vi "wd_replaceAll (WFM).vi"(7 "WFM":waveform(dbl), 8 "error in (no error)":errorcluster, 9 "channel index":i32, 10 "data type":T7, 11 "meta in":T1={"TargetFile"=path "", "StreamMode"=enum."File", "Append?"=FALSE, "ChunkSize"=0, "TimeColumnMode"=enum."Empty", "TimestampFormat"="", "AbsoluteTime?"=FALSE, "FileAttribute "={"Creator"="", "Title"="", "SheetName"=""}, "Column"=[], "FileRef"=refnum, "MemoryRef"=[], "RecordInfo"=[], " ChannelPreviousInfo"=[], "ChannelFirstRecord"=[], "PredefinedFormattedValueLength"=20, "DiskTemplate"={"XMLRef"=[refnum, refnum, refnum, refnum, refnum, refnum], "ZipPath"=path "", "MetaFile"={"Ref"=refnum, "NextRow"=0, "NextPosition"=0, "Block"=[]}, "TempFolder"=path ""}}) -> (0 "error out":errorcluster, 3 "meta out":T1={"TargetFile"=path "", "StreamMode"=enum."File", "Append?"=FALSE, "ChunkSize"=0, "TimeColumnMode"=enum."Empty", "TimestampFormat"="", "AbsoluteTime?"=FALSE, "FileAttribute "={"Creator"="", "Title"="", "SheetName"=""}, "Column"=[], "FileRef"=refnum, "MemoryRef"=[], "RecordInfo"=[], " ChannelPreviousInfo"=[], "ChannelFirstRecord"=[], "PredefinedFormattedValueLength"=20, "DiskTemplate"={"XMLRef"=[refnum, refnum, refnum, refnum, refnum, refnum], "ZipPath"=path "", "MetaFile"={"Ref"=refnum, "NextRow"=0, "NextPosition"=0, "Block"=[]}, "TempFolder"=path ""}})   [LabVIEW 2017, in "NI_ExcelFile.lvlib"]
uses:
  <vilib>/express/express shared/NI_ExcelFile/NI_ExcelFile.lvlib
  <vilib>/express/express shared/NI_ExcelFile/Ctrls/DataType.ctl
  <vilib>/express/express shared/NI_ExcelFile/Ctrls/MainData.ctl
  <vilib>/express/express shared/NI_ExcelFile/Ctrls/StreamMode.ctl
  <vilib>/express/express shared/NI_ExcelFile/Ctrls/TimeColumnMode.ctl
  <vilib>/express/express shared/NI_ExcelFile/Ctrls/FileAttribute.ctl
  <vilib>/express/express shared/NI_ExcelFile/Ctrls/Columns.ctl
  <vilib>/express/express shared/NI_ExcelFile/Ctrls/ColumnInfo.ctl
  <vilib>/express/express shared/NI_ExcelFile/Ctrls/wd_recordInfo.ctl
  <vilib>/express/express shared/NI_ExcelFile/Ctrls/disk_TemplateFile.ctl
  <vilib>/express/express shared/NI_ExcelFile/Ctrls/meta_file.ctl
  <vilib>/express/express shared/NI_ExcelFile/Ctrls/meta_Block.ctl
  <vilib>/express/express shared/NI_ExcelFile/Ctrls/meta_BlockType.ctl
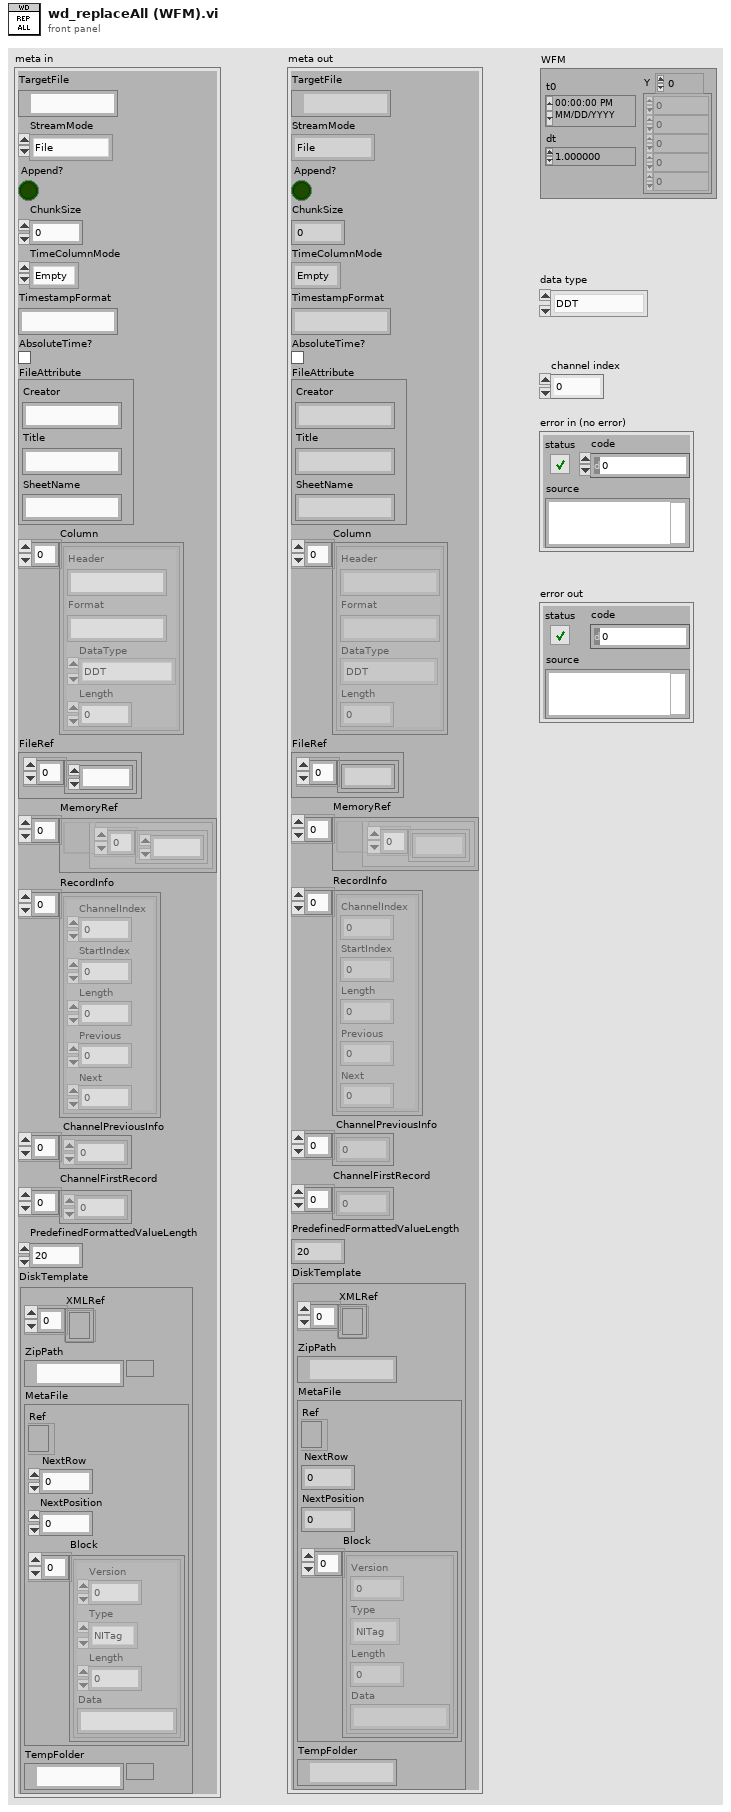
[diagram p1: front panel]
types:
  T1 = typedef "NI_ExcelFile.lvlib/MainData.ctl" = cluster{"TargetFile":path, "StreamMode":T2, "Append?":bool, "ChunkSize":u64, "TimeColumnMode":T3, "TimestampFormat":string, "AbsoluteTime?":bool, "FileAttribute ":T4, "Column":T5, "FileRef":refnum<k1>, "MemoryRef":refnum<data-value>[], "RecordInfo":T8[], " ChannelPreviousInfo":u32[], "ChannelFirstRecord":u32[], "PredefinedFormattedValueLength":i64, "DiskTemplate":T9}
  T2 = typedef "NI_ExcelFile.lvlib/StreamMode.ctl" = enum16{"File", "Memory"}
  T3 = typedef "NI_ExcelFile.lvlib/TimeColumnMode.ctl" = enum16{"Empty", "OnePerCh", "One"}
  T4 = typedef "NI_ExcelFile.lvlib/FileAttribute.ctl" = cluster{"Creator":string, "Title":string, "SheetName":string}
  T5 = typedef "NI_ExcelFile.lvlib/Columns.ctl" = T6[]
  T6 = typedef "NI_ExcelFile.lvlib/ColumnInfo.ctl" = cluster{"Header":string, "Format":string, "DataType":T7, "Length":u64}
  T7 = typedef "NI_ExcelFile.lvlib/DataType.ctl" = enum16{"DDT", "WFM", "Array of STR", "Array of DBL", "Array of I8", "Array of I16", "Array of I32", "Array of I64", "Array of SGL", "Array of U8", "Array of U16", "Array of U32", "Array of U64", "Array of Time"}
  T8 = typedef "NI_ExcelFile.lvlib/wd_recordInfo.ctl" = cluster{"ChannelIndex":u32, "StartIndex":u64, "Length":u64, "Previous":i32, "Next":i32}
  T9 = typedef "NI_ExcelFile.lvlib/disk_TemplateFile.ctl" = cluster{"XMLRef":refnum<file>[], "ZipPath":path, "MetaFile":T10, "TempFolder":path}
  T10 = typedef "NI_ExcelFile.lvlib/meta_file.ctl" = cluster{"Ref":refnum<file>, "NextRow":i32, "NextPosition":i64, "Block":T11[]}
  T11 = typedef "NI_ExcelFile.lvlib/meta_Block.ctl" = cluster{"Version":u16, "Type":T12, "Length":i32, "Data":string}
  T12 = typedef "NI_ExcelFile.lvlib/meta_BlockType.ctl" = enum16{"NITag", "File", "Column"}
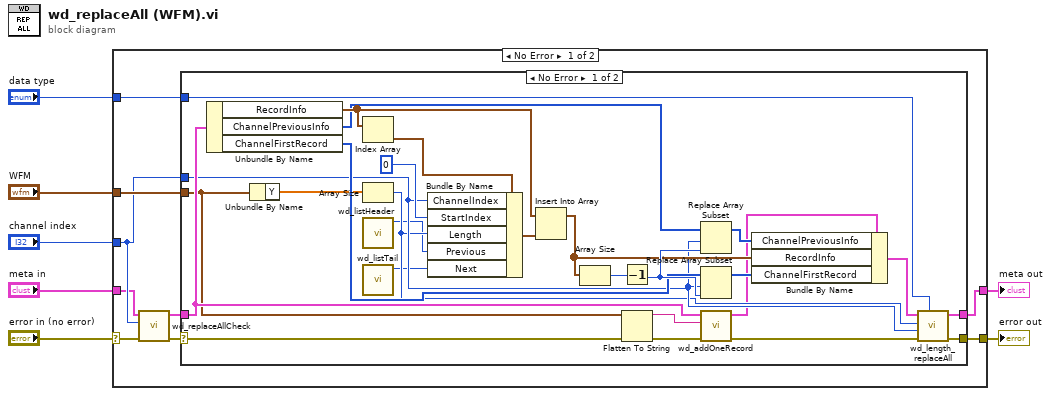
[diagram p0: block diagram]
diagram:
  n1 = case shown="No Error" "error in (no error)" {
    selector: "error in (no error)" -> [w8 w47]
    tunnel: "data type" -> [w13 _]
    tunnel: "channel index" -> [w12 _]
    tunnel: [w16 w46] -> w5
    tunnel: [w15 w47] -> w4
    tunnel: "WFM" -> [w14 _]
    tunnel: "meta in" -> [w11 w46]
    frame No Error {
      n2 = call <vilib>:"wd_replaceAllCheck.vi"("error in (no error)"=w8, "channel index"=w12, "meta in"=w11) -> ("error out"=w9:errorcluster, "meta out"=w10:T1)  [unwired: 7 in]
      n3 = case shown="No Error" w9 {
        selector: w9 -> [w23 w44]
        tunnel: [w24 w45] -> w16
        tunnel: [w21 w44] -> w15
        tunnel: w14 -> [w18 _]
        tunnel: w10 -> [w32 w45]
        tunnel: w13 -> [w27 _]
        tunnel: w12 -> [w29 _]
        frame No Error {
          n4 = Unbundle By Name(w32) -> ("RecordInfo"=w37:T8[], "ChannelPreviousInfo"=w34:u32[], "ChannelFirstRecord"=w33:u32[])
          n5 = Unbundle By Name(w18) -> ("Y"=w17:dbl[])
          n6 = Index Array(array=w37) -> (element=w35:T8)  [unwired: 1 in]
          n7 = Array Size(array=w17) -> (size(s)=w28:i32)
          n8 = call <vilib>:"wd_listHeader.vi"() -> ("list header"=w20:i32)  [unwired: 11 in]
          n9 = call <vilib>:"wd_listTail.vi"() -> ("list tail"=w19:i32)  [unwired: 11 in]
          n10 = Bundle By Name(cluster=w35, "ChannelIndex"=w29, "StartIndex"=u64 0 ("Start Index"), "Length"=w28, "Previous"=w20, "Next"=w19) -> (w38:T8)
          n11 = Insert Into Array(array=w37, new element=w38) -> (w41:T8[])  [unwired: 1 in]
          n12 = Array Size(array=w41) -> (size(s)=w39:i32)
          n13 = Decrement(x=w39) -> (x-1=w42:i32)
          n14 = Flatten To String(anything=w18, error in (no error)=w23) -> (data string=w31:string, error out=w30:errorcluster)  [unwired: 2 in, 1 out]
          n15 = Replace Array Subset(array=w34, new element=w42, index=w29) -> (w40:u32[])
          n16 = Replace Array Subset(array=w33, new element=w42, index=w29) -> (w43:u32[])
          n17 = call <vilib>:"wd_addOneRecord.vi"("error in (no error)"=w30, "data"=w31, "meta in"=w32) -> ("error out"=w22:errorcluster, "meta out"=w26:T1)  [unwired: 7 in]
          n18 = Bundle By Name(cluster=w26, "ChannelPreviousInfo"=w40, "RecordInfo"=w41, "ChannelFirstRecord"=w43) -> (w25:T1)
          n19 = call <vilib>:"wd_length_replaceAll.vi"("data type"=w27, "error in (no error)"=w22, "channel index"=w29, "size"=w28, "meta in"=w25) -> ("error out"=w21:errorcluster, "meta out"=w24:T1)  [unwired: 5 in]
        }
        frame Error {
        }
      }
    }
    frame Error {
    }
  }
  "error out" <- w4
  "meta out" <- w5
